vi "required keys.vi"() -> (3 "required keys":string[](array[string]))   [LabVIEW 2013]
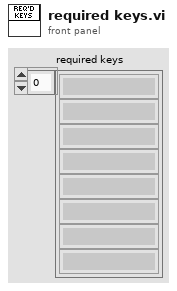
[diagram p1: front panel]
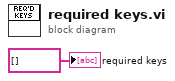
[diagram p0: block diagram]
diagram:
  "required keys" <- string[] [] ("required keys")
